vi "XML - Get relative Configuration LLB path.vi"(10 "CD Template":refnum<class "NIVS_CD Template.lvclass">, 11 "Project Name":string) -> (3 "Relative Configuration LLB path":path)   [LabVIEW 2015, in "NIVS_Consolidated_CDW_MetaDataObj.lvclass"]
doc: "Create the relative path for the Configuration LLB based on the name and execution mode of the new custom device."
uses:
  NIVS_Consolidated_CDW_MetaDataObj.lvclass
  Template Classes/NIVS_CD Template/NIVS_CD Template.lvclass
  Build Spec System Explorer.ctl
  Build Spec System Explorer.vi
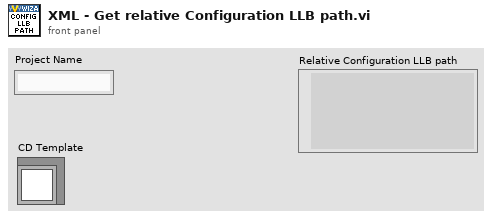
[diagram p1: front panel]
types:
  T1 = typedef "NIVS_Consolidated_CDW_MetaDataObj.lvclass/Build Spec System Explorer.ctl" = enum16{"Destinations.LLBFileName"}
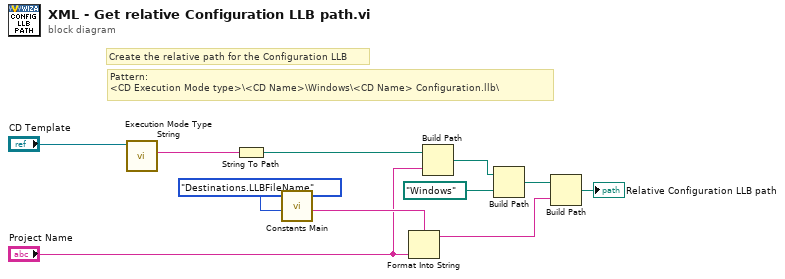
[diagram p0: block diagram]
diagram:
  # "Create the relative path for the Configuration LLB"
  # "Pattern:\n<CD Execution Mode type>\\<CD Name>\\Windows\\<CD Name> Configuration.llb\\"
  n1 = call-dynamic "Execution Mode Type String.vi"("CD Template"="CD Template") -> ("Execution Mode Type String"=w1:string)  [unwired: 10 in]
  n2 = String To Path(string=w1) -> (path=w7:path)
  n3 = call-poly "Constants Main.vi"("Action"=Build_Spec_System_Explorer."Destinations.LLBFileName") -> ("Output"=w9:string)  [unwired: 10 in]
  n4 = Format Into String(format string=w9, "Project Name") -> (resulting string=w10:string)  [unwired: 2 in, 1 out]
  n5 = Build Path(base path=w7, name or relative path="Project Name") -> (appended path=w6:path)
  n6 = Build Path(base path=w6, name or relative path=path "Windows") -> (appended path=w4:path)
  n7 = Build Path(base path=w4, name or relative path=w10) -> (appended path=→"Relative Configuration LLB path":path)
